vi "getPathArray.vi"(8 "Error In":errorcluster, 11 "File Path":path) -> (0 "Error Out":errorcluster, 2 "Folder Path Array":path[](array[path]), 3 "File Path Array":path[](array[path]))   [LabVIEW 2018]
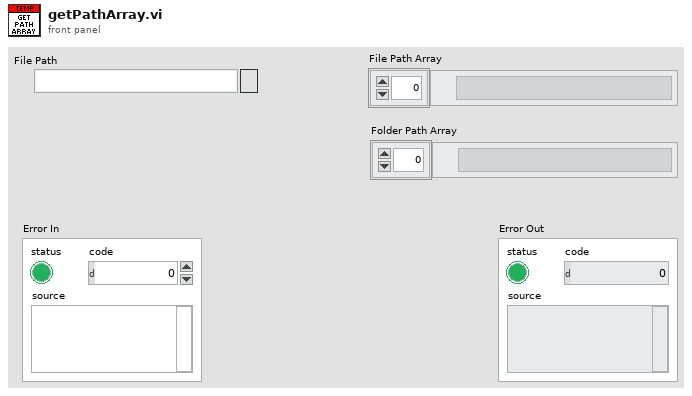
[diagram p1: front panel]
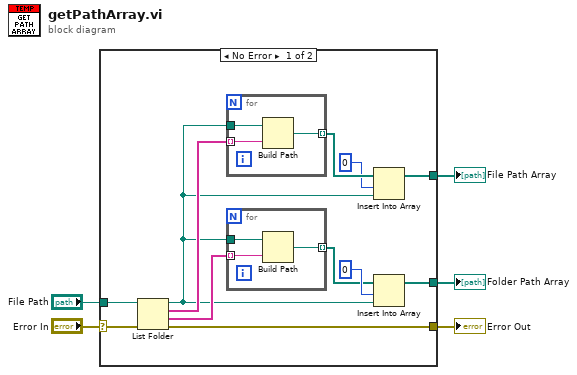
[diagram p0: block diagram]
diagram:
  n1 = case shown="No Error" "Error In" {
    selector: "Error In" -> [w13 w24]
    tunnel: "File Path" -> [w17 _]
    tunnel: [w12 w24] -> w1
    tunnel: [w14 _] -> w3
    tunnel: [w6 _] -> w2
    frame No Error {
      n2 = List Folder(path=w17, error in=w13) -> (path out=w8:path, filenames=w10:string[], folder names=w11:string[], error out=w12:errorcluster)  [unwired: 2 in]
      n3 = for {
        tunnel: w10 -> [w22] mode=indexing
        tunnel: w8 -> [w23]
        tunnel: [w21] -> w16 mode=indexing
        n4 = Build Path(base path=w23, name or relative path=w22) -> (appended path=w21:path)
      }
      n5 = for {
        tunnel: w11 -> [w19] mode=indexing
        tunnel: w8 -> [w20]
        tunnel: [w18] -> w7 mode=indexing
        n6 = Build Path(base path=w20, name or relative path=w19) -> (appended path=w18:path)
      }
      n7 = Insert Into Array(array=w16, index=0, new element=w8) -> (w14:path[])
      n8 = Insert Into Array(array=w7, index=0, new element=w8) -> (w6:path[])
    }
    frame Error {
    }
  }
  "File Path Array" <- w3
  "Error Out" <- w1
  "Folder Path Array" <- w2
